vi "turnAround_v3.vi"(6 "Center":dbl[](array[numeric]), 8 "error in (no error)":errorcluster, 9 "clockwise?":bool, 10 "Robot":refnum<class "Robot.lvclass">, 11 "KickToSkill in":refnum<class "KickToSkill.lvclass">) -> (0 "error out":errorcluster, 2 "Robot out":refnum<class "Robot.lvclass">, 3 "KickToSkill out":refnum<class "KickToSkill.lvclass">)   [LabVIEW 2023, in "KickToSkill.lvclass"]
uses:
  KickToSkill.lvclass
  Robot_class/Robot.lvclass
  Game_class/Navigation/driveMode.ctl
  Robot_class/robotKickToStates.ctl
  Robot_class/Robot.lvclass/Robot.ctl
  Robot_class/Write robotKickState.vi
  Robot_class/Write dest_x.vi
  Robot_class/Write dest_y.vi
  Robot_class/Write dest_orientation.vi
  Utilities_class/Utilities.lvclass
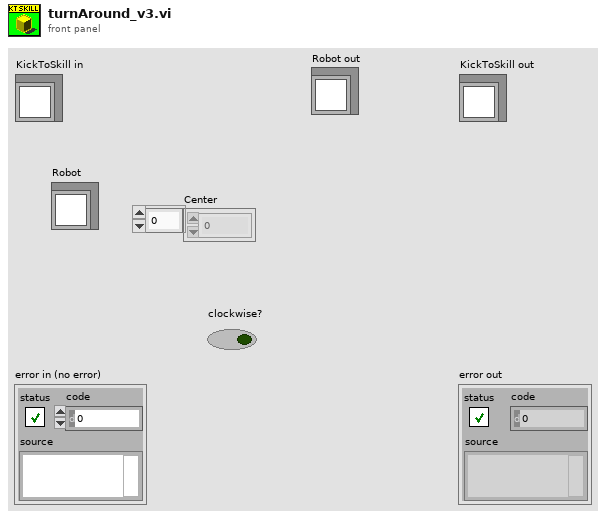
[diagram p1: front panel]
types:
  T1 = typedef "robotKickToStates.ctl" = enum16{"shootFromDirect", "avoidCollideBall", "goToBackBall", "none", "walk", "turnAntiClockwise", "turnClockwise", "oldKickToShoot", "oldKickToGoToBackBall", "shoot"}
  T2 = typedef "driveMode.ctl" = enum16{"Fast", "SafeDrive"}
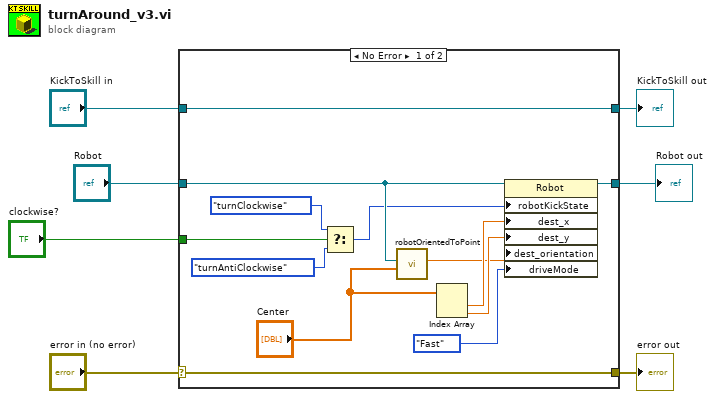
[diagram p0: block diagram]
diagram:
  n1 = case shown="No Error" "error in (no error)" {
    selector: "error in (no error)" -> [w19 w23]
    tunnel: [w19 w23] -> w6
    tunnel: [w20 w22] -> w4
    tunnel: "KickToSkill in" -> [w20 w22]
    tunnel: "Robot" -> [w14 w21]
    tunnel: [w18 w21] -> w2
    tunnel: "clockwise?" -> [w11 _]
    frame No Error {
      n2 = Select(t=robotKickToStates."turnClockwise" ("robotKickState"), s=w11, f=robotKickToStates."turnAntiClockwise" ("robotKickState")) -> (s? t:f=w8:T1)
      n3 = call "robotOrientedToPoint.vi"("Target"="Center", "Robot"=w14) -> ("Orientation"=w13:dbl)  [unwired: 7 in, 2 out]
      n4 = Index Array(array="Center") -> (element #1=w16:dbl, element #2=w15:dbl)  [unwired: 2 in]
      n5 = property class="Robot"(reference=w14, "robotKickState"=w8, "dest_x"=w16, "dest_y"=w15, "dest_orientation"=w13, "driveMode"=driveMode."Fast") -> (reference out=w18:refnum<class "Robot.lvclass">)  [unwired: 1 in, 1 out]
    }
    frame Error {
    }
  }
  "error out" <- w6
  "KickToSkill out" <- w4
  "Robot out" <- w2
